vi "ActionVIOnCompile.vi"(8 "error in (no error)":errorcluster, 11 "Device Item Ref in":T2 format="%.0x") -> (0 "error out":errorcluster)   [LabVIEW 2015, in "SLSC-12201 DIO System Explorer.lvlib"]
uses:
  SLSC-12201 DIO System Explorer.lvlib
  <vilib>/NI Veristand/Custom Device API/Custom Device Item Ref.ctl
  Shared/SLSC Dynamic Channel.ctl
  Shared/SLSC Dynamic Channel Type.ctl
  Shared/Compiled.Settings
  Shared/Constants.vi
  <vilib>/NI Veristand/Custom Device Tools/Custom Device Utility Library/NI VeriStand - Search for Item by Name.vi
  <vilib>/NI Veristand/Custom Device API/Get Item Property (I32).vi
  <vilib>/NI Veristand/Custom Device API/Get Item Property (U32).vi
  <vilib>/NI Veristand/Custom Device API/Get Item Property (String).vi
  <vilib>/NI Veristand/Custom Device Tools/Custom Device Utility Library/NI VeriStand - Search for All Items by Name.vi
  <vilib>/NI Veristand/Custom Device API/Set Item Property (Variant).vi
  <vilib>/NI Veristand/Custom Device Tools/Custom Device Utility Library/Custom Device Utility Library.lvlib
  <vilib>/NI Veristand/Custom Device API/Custom Device API.lvlib
  <vilib>/NI/NIVS Inline Async API/_Data Access System Explorer/Data Access System Explorer.lvlib
  Shared/SLSC-12201 DIO Shared.lvlib
panel:
  out "appended array 2":T1(array[cluster]) {"Dev.ProductNumber" format="%.0x"; "Dev.VendorNumber" format="%.0x"}
  out "appended array":T3(array[cluster]) {"VS Refs" format="%.0x"}
  out "SLSC Commands":T4[](array[typedef])
  out "SLSC Set/Write Properties":T4[](array[typedef])
  out "SLSC Get/Read Properties":T4[](array[typedef])
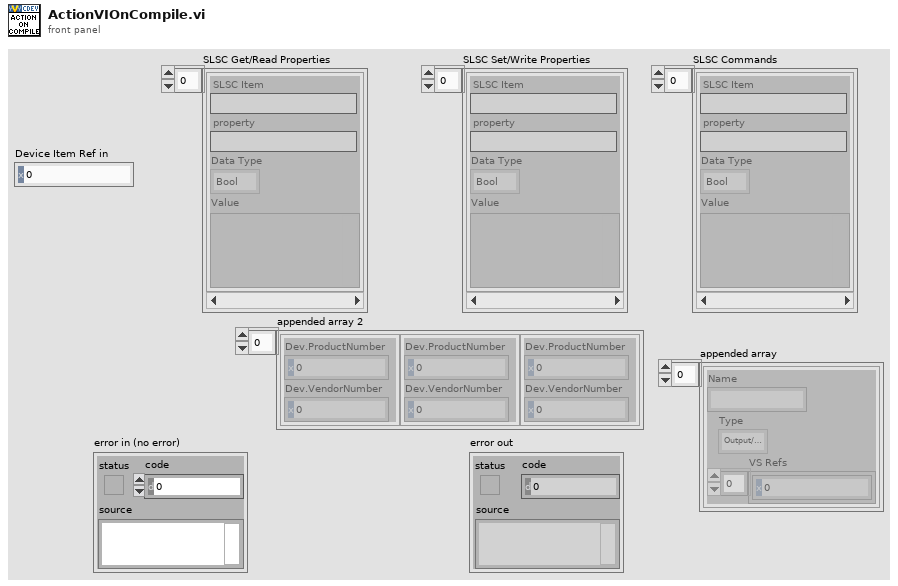
[diagram p1: front panel]
types:
  T1 = cluster{"Dev.ProductNumber":u32, "Dev.VendorNumber":u32}[]
  T2 = typedef "Custom Device API.lvlib/Custom Device Item Ref.ctl" = u64
  T3 = cluster{"Name":string, "Type":enum16{"Output/Write", "Input/Read", "Input/ReadWrite"}, "VS Refs":T2[]}[]
  T4 = typedef "SLSC-12201 DIO System Explorer.lvlib/SLSC Dynamic Channel.ctl" = cluster{"SLSC Item":string, "property":string, "Data Type":T5, "Value":variant}
  T5 = typedef "SLSC-12201 DIO System Explorer.lvlib/SLSC Dynamic Channel Type.ctl" = enum16{"Bool", "Double", "I32", "I64", "String", "U32", "U64", "EnumI32"}
  T6 = cluster{"Dev.ProductNumber":u32, "Dev.VendorNumber":u32}
  T7 = enum16{"Output/Write", "Input/Read", "Input/ReadWrite"}
  T8 = typedef "SLSC-12201 DIO Shared.lvlib/Compiled.Settings" = cluster{"Name":string, "SLSC IP Address":string, "Slot #":i32, "Configuration Data":cluster{"Properties":cluster{"Boolean Properties":cluster{"property":refnum<k21>, "Value":bool, "SLSC Item":refnum<k21>}[], "Double Properties":cluster{"property":refnum<k21>, "Double Write":dbl, "SLSC Item":refnum<k21>}[], "I32 Properties":cluster{"property":refnum<k21>, "Int32 Write":i32, "SLSC Item":refnum<k21>}[], "I64 Properties":cluster{"property":refnum<k21>, "Int64 Write":i64, "SLSC Item":refnum<k21>}[], "String Properties":cluster{"property":refnum<k21>, "String Write":string, "SLSC Item":refnum<k21>}[], "U32 Properties":cluster{"property":refnum<k21>, "UInt32 Write":u32, "SLSC Item":refnum<k21>}[], "U64 Properties":cluster{"property":refnum<k21>, "UInt64 Write":u64, "SLSC Item":refnum<k21>}[]}}, "SLSC Set Properties":T4[], "SLSC Get Properties":T4[], "SLSC Commands":T4[], "Username":string, "Password":string, "Support Modules":cluster{"Dev.ProductNumber":u32, "Dev.VendorNumber":u32}[]}
  T9 = cluster{"Name":string, "Type":enum16{"Output/Write", "Input/Read", "Input/ReadWrite"}, "VS Refs":T2[]}
  T10 = typedef "Custom Device API.lvlib/Custom Device Item Info.ctl" = cluster{"Name":string, "Is Channel":bool, "GUID":string, "Is Waveform":bool}
  T11 = cluster{"Properties":cluster{"Boolean Properties":cluster{"property":refnum<k21>, "Value":bool, "SLSC Item":refnum<k21>}[], "Double Properties":cluster{"property":refnum<k21>, "Double Write":dbl, "SLSC Item":refnum<k21>}[], "I32 Properties":cluster{"property":refnum<k21>, "Int32 Write":i32, "SLSC Item":refnum<k21>}[], "I64 Properties":cluster{"property":refnum<k21>, "Int64 Write":i64, "SLSC Item":refnum<k21>}[], "String Properties":cluster{"property":refnum<k21>, "String Write":string, "SLSC Item":refnum<k21>}[], "U32 Properties":cluster{"property":refnum<k21>, "UInt32 Write":u32, "SLSC Item":refnum<k21>}[], "U64 Properties":cluster{"property":refnum<k21>, "UInt64 Write":u64, "SLSC Item":refnum<k21>}[]}}
  T12 = typedef "Custom Device API.lvlib/Custom Device Channel.ctl" = cluster{"Type":T13, "Units":string, "Default Value":dbl, "Faultable":bool, "Scalable":bool}
  T13 = typedef "Custom Device API.lvlib/Custom Device Channel Type.ctl" = enum16{"Input", "Output"}
  T14 = cluster{"Channel Name":string, "SLSC Name":string, "Channel":T12}[]
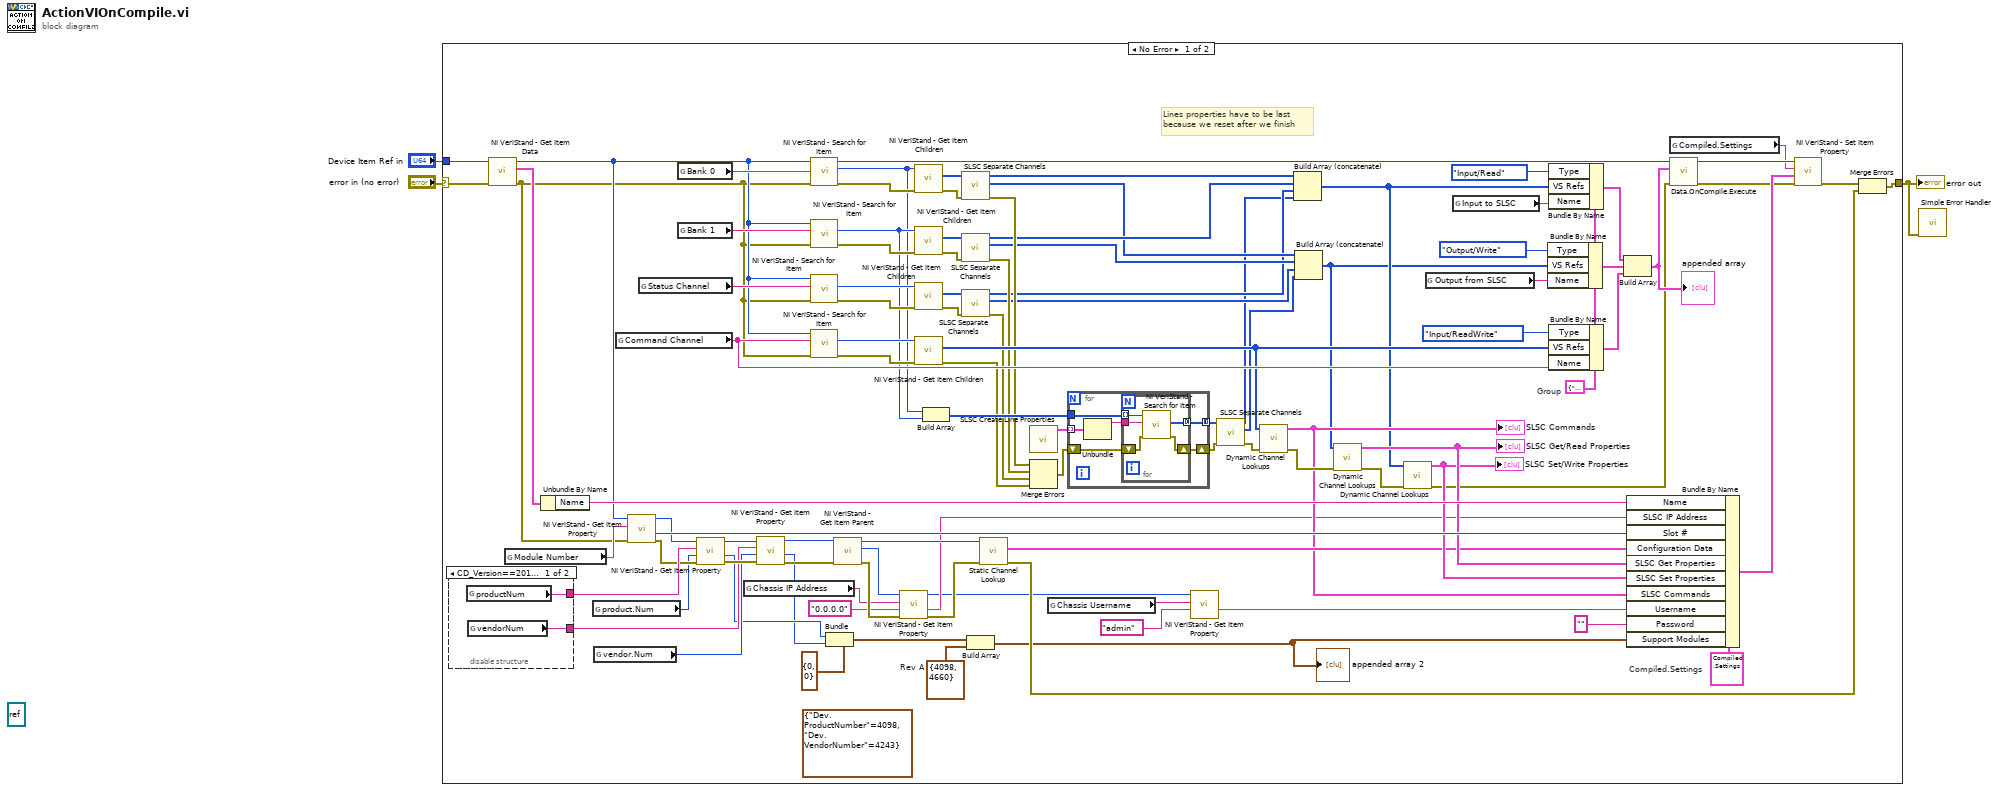
[diagram p0: block diagram]
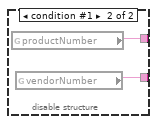
[diagram p2: hidden frame]
diagram:
  (unwired) refnum<k7> refnum ("SHDocVw.IWebBrowser2")
  n1 = case shown="No Error" "error in (no error)" {
    selector: "error in (no error)" -> [w89 w120]
    tunnel: [w87 w120] -> w1
    tunnel: "Device Item Ref in" -> [w90 _]
    frame No Error {
      (unwired) T6 {"Dev.ProductNumber"=4098, "Dev.VendorNumber"=4243} ("element")
      w9 = T6 {"Dev.ProductNumber"=4098, "Dev.VendorNumber"=4660}  # Rev A
      w80 = T8 {"Name"="", "SLSC IP Address"="", "Slot #"=0, "Configuration Data"={"Properties"={"Boolean Properties"=[], "Double Properties"=[], "I32 Properties"=[], "I64 Properties"=[], "String Properties"=[], "U32 Properties"=[], "U64 Properties"=[]}}, "SLSC Set Properties"=[], "SLSC Get Properties"=[], "SLSC Commands"=[], "Username"="admin", "Password"="", "Support Modules"=[]}  # Compiled.Settings
      w45 = T9 {"Name"="", "Type"=enum."Output/Write", "VS Refs"=[]}  # Group
      # "Lines properties have to be last\nbecause we reset after we finish"
      n2 = disable-structure shown="CD_Version==2015_2016" {
        disable-tunnel: [w106 w108] -> w61
        disable-tunnel: [w105 w107] -> w13
        frame condition #0 (active) {
          n3 = global read "Constants.vi" "productNum"() -> (w106:string)
          n4 = global read "Constants.vi" "vendorNum"() -> (w105:string)
        }
        frame condition #1 {
          n5 = global read "Constants.vi" "productNumber"() -> (w108:string)
          n6 = global read "Constants.vi" "vendorNumber"() -> (w107:string)
        }
      }
      n7 = call <vilib>:"NI VeriStand - Get Item Data.vi"("error in (no error)"=w89, "Item Ref in"=w90) -> ("error out"=w42:errorcluster, "Item Info"=w102:T10, "Item Ref out"=w43:T2)  [unwired: 6 in, 1 out]
      n8 = global read "Constants.vi" "Module Number"() -> (w92:string)
      n9 = Unbundle By Name(w102) -> ("Name"=w101:string)
      n10 = global read "Constants.vi" "product.Num"() -> (w53:i32)
      n11 = global read "Constants.vi" "vendor.Num"() -> (w12:i32)
      n12 = global read "Constants.vi" "Command Channel"() -> (w69:string)
      n13 = call-poly <vilib>:"NI VeriStand - Get Item Property.vi"("error in (no error)"=w42, "Property Name"=w92, "Item Ref in"=w43) -> ("error out"=w59:errorcluster, "Value"=w93:i32, "Item Ref out"=w60:T2)  [unwired: 5 in, 1 out]
      n14 = global read "Constants.vi" "Status Channel"() -> (w75:string)
      n15 = global read "Constants.vi" "Bank 0"() -> (w83:string)
      n16 = global read "Constants.vi" "Bank 1"() -> (w51:string)
      n17 = call-poly <vilib>:"NI VeriStand - Get Item Property.vi"("error in (no error)"=w59, "Default Value"=w53, "Property Name"=w61, "Item Ref in"=w60) -> ("error out"=w14:errorcluster, "Value"=w7:u32, "Item Ref out"=w17:T2)  [unwired: 4 in, 1 out]
      n18 = global read "Constants.vi" "Chassis IP Address"() -> (w91:string)
      n19 = call-poly <vilib>:"NI VeriStand - Get Item Property.vi"("error in (no error)"=w14, "Default Value"=w12, "Property Name"=w13, "Item Ref in"=w17) -> ("error out"=w15:errorcluster, "Value"=w6:u32, "Item Ref out"=w16:T2)  [unwired: 4 in, 1 out]
      n20 = call-poly <vilib>:"NI VeriStand - Search for Item.vi"("error in"=w42, "Item Name"=w83, "Section Ref in"=w43) -> ("error out"=w74:errorcluster, "Item Ref"=w32:T2, "Section Ref out"=w31:T2)  [unwired: 5 in, 1 out]
      n21 = call-poly <vilib>:"NI VeriStand - Search for Item.vi"("error in"=w42, "Item Name"=w51, "Section Ref in"=w43) -> ("error out"=w85:errorcluster, "Item Ref"=w47:T2)  [unwired: 5 in, 2 out]
      n22 = call-poly <vilib>:"NI VeriStand - Search for Item.vi"("error in"=w42, "Item Name"=w75, "Section Ref in"=w43) -> ("error out"=w76:errorcluster, "Item Ref"=w58:T2)  [unwired: 5 in, 2 out]
      n23 = call-poly <vilib>:"NI VeriStand - Search for Item.vi"("error in"=w42, "Item Name"=w69, "Section Ref in"=w43) -> ("error out"=w71:errorcluster, "Item Ref"=w72:T2)  [unwired: 5 in, 2 out]
      n24 = Bundle(cluster=T6 {"Dev.ProductNumber"=0, "Dev.VendorNumber"=0} ("Product Identification"), "Dev.ProductNumber"=w7, "Dev.VendorNumber"=w6) -> (w8:T6)
      n25 = call <vilib>:"NI VeriStand - Get Item Parent.vi"("error in (no error)"=w15, "Item Ref in"=w16) -> ("error out"=w95:errorcluster, "Parent Ref"=w94:T2, "Item Ref out"=w77:T2)  [unwired: 6 in, 1 out]
      n26 = call-poly <vilib>:"NI VeriStand - Get Item Property.vi"("error in (no error)"=w95, "Default Value"="0.0.0.0", "Property Name"=w91, "Item Ref in"=w94) -> ("error out"=w78:errorcluster, "Value"=w64:string, "Item Ref out"=w55:T2)  [unwired: 4 in, 1 out]
      n27 = call <vilib>:"NI VeriStand - Get Item Children.vi"("error in (no error)"=w74, "Item Ref in"=w32) -> ("error out"=w39:errorcluster, "Child Refs"=w44:T2[])  [unwired: 6 in, 2 out]
      n28 = call <vilib>:"NI VeriStand - Get Item Children.vi"("error in (no error)"=w85, "Item Ref in"=w47) -> ("error out"=w38:errorcluster, "Child Refs"=w49:T2[])  [unwired: 6 in, 2 out]
      n29 = call <vilib>:"NI VeriStand - Get Item Children.vi"("error in (no error)"=w76, "Item Ref in"=w58) -> ("error out"=w37:errorcluster, "Child Refs"=w46:T2[])  [unwired: 6 in, 2 out]
      n30 = call <vilib>:"NI VeriStand - Get Item Children.vi"("error in (no error)"=w71, "Item Ref in"=w72) -> ("error out"=w33:errorcluster, "Child Refs"=w66:T2[])  [unwired: 6 in, 2 out]
      n31 = Build Array(w32, w47) -> (w48:T2[])
      n32 = call "SLSC Separate Channels.vi"("error in (no error)"=w39, "Item Refs In"=w44) -> ("error out"=w34:errorcluster, "Output Channels"=w28:T2[], "Input Channels"=w30:T2[])  [unwired: 6 in, 1 out]
      n33 = call "SLSC Separate Channels.vi"("error in (no error)"=w38, "Item Refs In"=w49) -> ("error out"=w35:errorcluster, "Output Channels"=w27:T2[], "Input Channels"=w29:T2[])  [unwired: 6 in, 1 out]
      n34 = call "SLSC Separate Channels.vi"("error in (no error)"=w37, "Item Refs In"=w46) -> ("error out"=w36:errorcluster, "Output Channels"=w26:T2[], "Input Channels"=w5:T2[])  [unwired: 6 in, 1 out]
      n35 = Build Array(w8, w9) -> (w11:T1)
      "appended array 2" <- w11
      n36 = call "Static Channel Lookup.vi"("error in (no error)"=w78, "Device Item Ref in"=w77) -> ("error out"=w73:errorcluster, "Configuration Data"=w79:T11)  [unwired: 7 in, 1 out]
      n37 = call "SLSC Create Line Properties.vi"() -> ("Outgoing configuration"=w50:T14)  [unwired: 11 in]
      n38 = Merge Errors(w34, w35, w36, w33) -> (w41:errorcluster)
      n39 = global read "Constants.vi" "Chassis Username"() -> (w56:string)
      n40 = for {
        tunnel: w50 -> [w114] mode=indexing
        tunnel: [w112] -> w23 mode=concatenating
        shift-right: [w110] -> w19
        shift-left: w41 -> [w111]
        tunnel: w48 -> [w109]
        n41 = Unbundle(w114) -> ("Channel Name"=w113:string)  [unwired: 2 out]
        n42 = for {
          tunnel: w113 -> [w119]
          tunnel: [w118] -> w112 mode=concatenating
          tunnel: w109 -> [w115] mode=indexing
          shift-right: [w116] -> w110
          shift-left: w111 -> [w117]
          n43 = call-poly <vilib>:"NI VeriStand - Search for Item.vi"("error in"=w117, "Item Name"=w119, "Section Ref in"=w115) -> ("error out"=w116:errorcluster, "Item Refs"=w118:T2[])  [unwired: 5 in, 2 out]
        }
      }
      n44 = call-poly <vilib>:"NI VeriStand - Get Item Property.vi"("Default Value"="admin", "Property Name"=w56, "Item Ref in"=w55) -> ("Value"=w54:string)  [unwired: 5 in, 3 out]
      n45 = call "SLSC Separate Channels.vi"("error in (no error)"=w19, "Item Refs In"=w23) -> ("error out"=w18:errorcluster, "Output Channels"=w22:T2[], "Input Channels"=w4:T2[])  [unwired: 6 in, 1 out]
      n46 = call "Dynamic Channel Lookups.vi"("error in (no error)"=w18, "Child Refs"=w66) -> ("error out"=w67:errorcluster, "SLSC Dynamic Inputs"=w65:T4[])  [unwired: 8 in]
      "SLSC Commands" <- w65
      n47 = Build Array (concatenate)(w30, w29, w5, w4) -> (w21:T2[])
      n48 = Build Array (concatenate)(w28, w27, w26, w22) -> (w20:T2[])
      n49 = call "Dynamic Channel Lookups.vi"("error in (no error)"=w67, "Child Refs"=w20) -> ("error out"=w84:errorcluster, "SLSC Dynamic Inputs"=w86:T4[])  [unwired: 8 in]
      "SLSC Get/Read Properties" <- w86
      n50 = call "Dynamic Channel Lookups.vi"("error in (no error)"=w84, "Child Refs"=w21) -> ("error out"=w40:errorcluster, "SLSC Dynamic Inputs"=w81:T4[])  [unwired: 8 in]
      "SLSC Set/Write Properties" <- w81
      n51 = global read "Constants.vi" "Output from SLSC"() -> (w82:string)
      n52 = global read "Constants.vi" "Input to SLSC"() -> (w52:string)
      n53 = Bundle By Name(cluster=w45, "Type"=T7."Output/Write", "VS Refs"=w20, "Name"=w82) -> (w24:T9)
      n54 = Bundle By Name(cluster=w45, "Type"=T7."Input/Read", "VS Refs"=w21, "Name"=w52) -> (w25:T9)
      n55 = Bundle By Name(cluster=w45, "Type"=T7."Input/ReadWrite", "VS Refs"=w66, "Name"=w69) -> (w68:T9)
      n56 = Build Array(w25, w24, w68) -> (w99:T3)
      "appended array" <- w99
      n57 = Bundle By Name(cluster=w80, "Name"=w101, "SLSC IP Address"=w64, "Slot #"=w93, "Configuration Data"=w79, "SLSC Get Properties"=w86, "SLSC Set Properties"=w81, "SLSC Commands"=w65, "Username"=w54, "Password"="", "Support Modules"=w11) -> (w104:T8)
      n58 = global read "Constants.vi" "Compiled.Settings"() -> (w88:string)
      n59 = call <vilib>:"Data.OnCompile.Execute.vi"("error in"=w40, "VS Ref Groups"=w99, "Custom Device Ref"=w31) -> ("error out"=w97:errorcluster, "Custom Device Ref"=w96:T2)  [unwired: 7 in]
      n60 = call-poly <vilib>:"NI VeriStand - Set Item Property.vi"("error in (no error)"=w97, "Value"=w104, "Property Name"=w88, "Item Ref in"=w96) -> ("error out"=w103:errorcluster)  [unwired: 5 in, 2 out]
      n61 = Merge Errors(w103, w73) -> (w87:errorcluster)
    }
    frame Error {
    }
  }
  "error out" <- w1
  n62 = call <vilib>:"Simple Error Handler.vi"("error in (no error)"=w1) -> ()  [unwired: 4 in, 5 out]
